vi "Test_Cmd_n.vi"(8 "error in":errorcluster, 11 "Port?":string="COM1") -> (0 "error out":errorcluster)   [LabVIEW 2016, in "Serial_G.lvlib"]
doc: "Tests an array of cmds at a time"
uses:
  Serial_G.lvlib
  Controls/Cmd_Tx.ctl
  Controls/Cmd_Rx.ctl
  Controls/PortConfig.ctl
panel:
  in  "Log?":bool
  in  "Delay(ms)":u32=50
  out "Responses":T1[](array[typedef])
  in  "Cmds":T2[](array[typedef])
  out "Port?":bool
  # "Serial Communication Driver - Commands array"
  # "Cmd                                                                   w/Read?"
  # "Response                                                            Exec time   Timeout?"
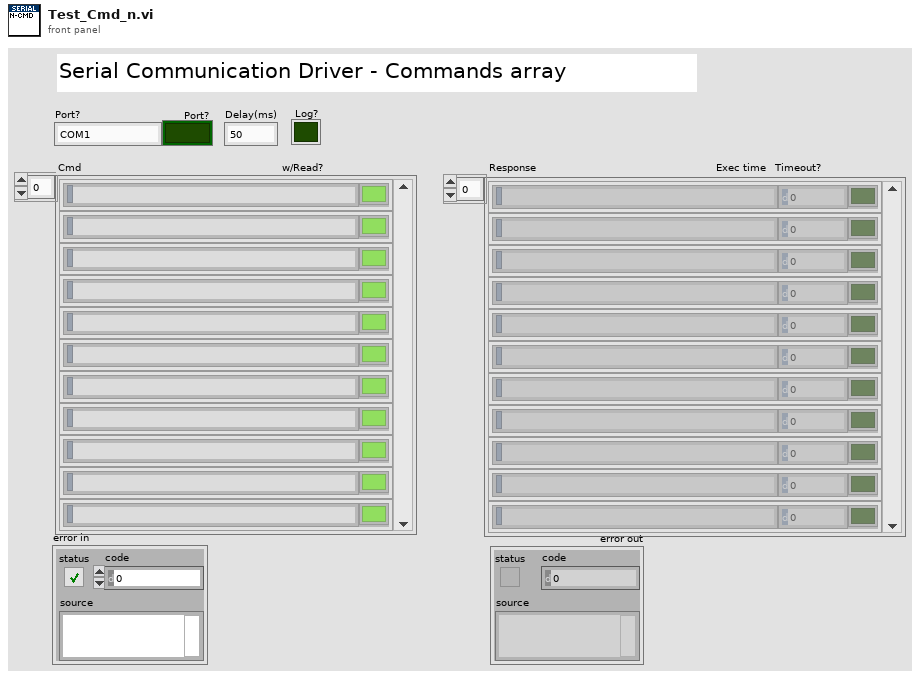
[diagram p1: front panel]
types:
  T1 = typedef "Serial_G.lvlib/Cmd_Rx.ctl" = cluster{"Read":string, "ExecTime (ms)":i32, "Timeout?":bool}
  T2 = typedef "Serial_G.lvlib/Cmd_Tx.ctl" = cluster{"Write":string, "Fbk?":bool}
  T3 = typedef "Serial_G.lvlib/PortConfig.ctl" = cluster{"Baud rate":u32, "Parity":enum16{"None", "Odd", "Even", "Mark", "Space"}, "Data bits":u16, "Stop bits":u16, "Flow control":u16}
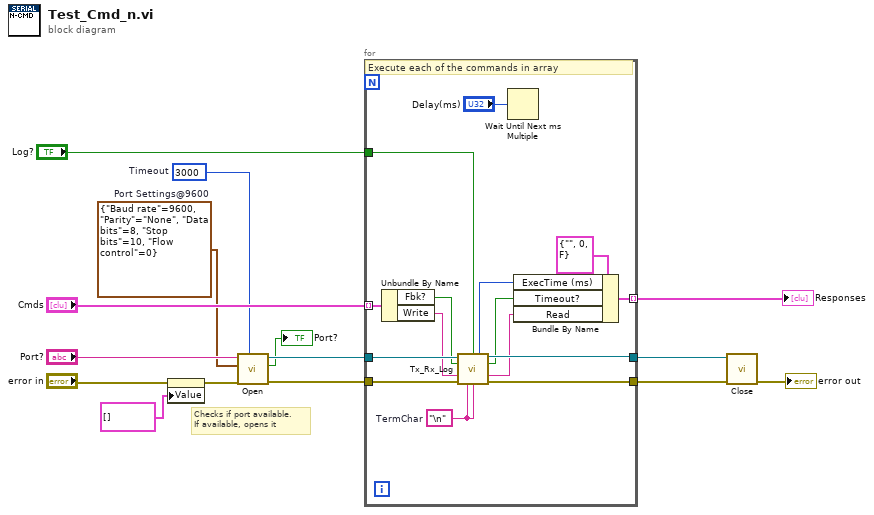
[diagram p0: block diagram]
diagram:
  w1 = u32 3000  # Timeout
  w3 = T3 {"Baud rate"=9600, "Parity"=enum."None", "Data bits"=8, "Stop bits"=10, "Flow control"=0}  # Port Settings@9600
  # "Checks if port available.\nIf available, opens it"
  n1 = property on="Responses" class="Arr (strict)"(error in="error in", "Value"=T1[] [] ("Responses")) -> (error out=w5:errorcluster)  [unwired: 1 in, 1 out]
  n2 = call "Open.vi"("Timeout (3000)"=w1, "error in"=w5, "ConfigPort (9600,0,8,1)"=w3, "Port(Alias)"="Port?") -> ("error out"=w15:errorcluster, "PortFound?"=→"Port?":bool, "VISA out"=w14:refnum<visa-resource-name>)  [unwired: 4 in, 1 out]
  n3 = for {
    tunnel: "Cmds" -> [w25] mode=indexing
    tunnel: [w17] -> w7 mode=indexing
    tunnel: "Log?" -> [w16]
    tunnel: w15 -> [w30]
    tunnel: [w27] -> w11
    tunnel: w14 -> [w29]
    tunnel: [w28] -> w13
    w26 = "\n"  # TermChar
    # "Execute each of the commands in array"
    n4 = Unbundle By Name(w25) -> ("Fbk?"=w23:bool, "Write"=w24:string)
    n5 = call "Tx_Rx_Log.vi"("VISA in"=w29, "Log?"=w16, "Fbk? (T)"=w23, "Write"=w24, "error in"=w30, "TermChar (\\n)"=w26, "Wait for? (\\n)"=w26) -> ("ExecTime(ms)"=w20:i32, "VISA out"=w28:refnum<visa-resource-name>, "Timeout?"=w19:bool, "Read"=w18:string, "error out"=w27:errorcluster)  [unwired: 4 in]
    n6 = Wait Until Next ms Multiple(millisecond multiple="Delay(ms)") -> ()  [unwired: 1 out]
    n7 = Bundle By Name(cluster=T1 {"Read"="", "ExecTime (ms)"=0, "Timeout?"=FALSE} ("Read"), "ExecTime (ms)"=w20, "Timeout?"=w19, "Read"=w18) -> (w17:T1)
  }
  "Responses" <- w7
  n8 = call "Close.vi"("error in"=w11, "VISA in"=w13) -> ("error out"=→"error out":errorcluster)  [unwired: 9 in]
